vi "Check_Subtrack_Length-1.vi"(2 "[IN] Subtrack":T1, 3 "[IN] Minimal Sub\ntrack Length":i32) -> (0 "[OUT] Subtrack":T1)   [LabVIEW 2017]
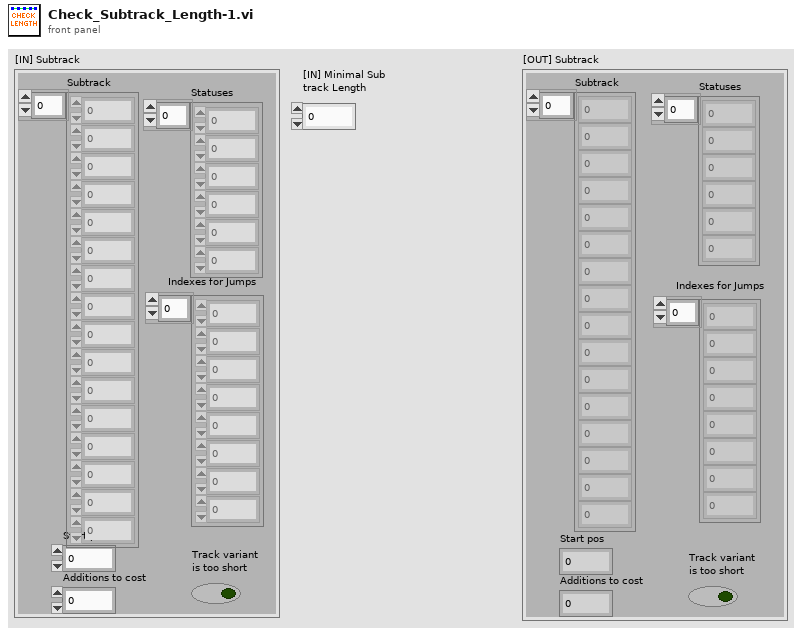
[diagram p1: front panel]
types:
  T1 = cluster{"Subtrack":dbl[], "Statuses":i16[], "Start pos":i32, "Additions to cost":i8, "Track variant \nis too short":bool, "Indexes for Jumps":i32[]}
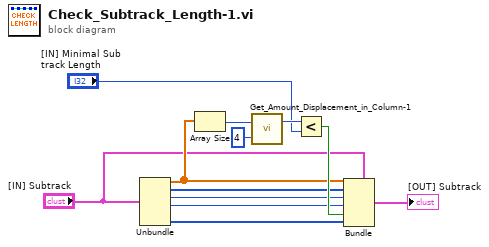
[diagram p0: block diagram]
diagram:
  n1 = Unbundle("[IN] Subtrack") -> ("Subtrack"=w7:dbl[], "Statuses"=w8:i16[], "Start pos"=w6:i32, "Additions to cost"=w5:i8, "Indexes for Jumps"=w4:i32[])  [unwired: 1 out]
  n2 = Array Size(array=w7) -> (size(s)=w12:i32)
  n3 = call "Get_Amount_Displacement_in_Column-1.vi"("multiplier"=4, "# Rows"=w12) -> ("Displ amount"=w11:i32)  [unwired: 1 out]
  n4 = Less?(x=w11, y="[IN] Minimal Sub\ntrack Length") -> (x < y?=w9:bool)
  n5 = Bundle(cluster="[IN] Subtrack", "Subtrack"=w7, "Statuses"=w8, "Start pos"=w6, "Additions to cost"=w5, "Track variant \nis too short"=w9, "Indexes for Jumps"=w4) -> (→"[OUT] Subtrack":T1)
